vi "4.4.vi"() -> ()   [LabVIEW 2016]
panel:
  out "数组":i32[][](array[numeric])
  out "强度图":i32[][](graph)
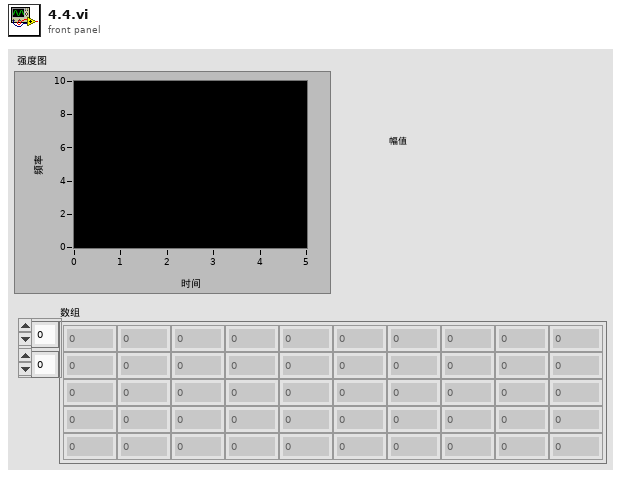
[diagram p1: front panel]
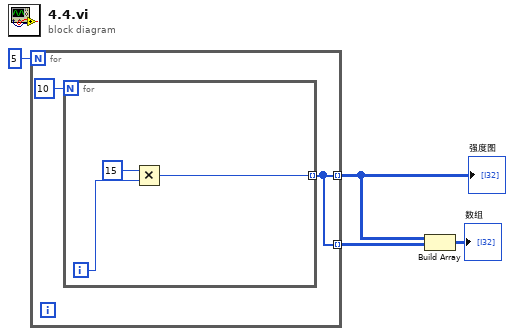
[diagram p0: block diagram]
diagram:
  n1 = for {
    N: 5 -> [_]
    tunnel: [w5] -> w2 mode=indexing
    tunnel: [w5] -> w3 mode=indexing
    n2 = for {
      N: 10 -> [_]
      tunnel: [w7] -> w5 mode=indexing
      i -> [w9]
      n3 = Multiply(x=15, y=w9) -> (x*y=w7:i32)
    }
  }
  "强度图" <- w2
  n4 = Build Array(w2, w3) -> (→"数组":i32[][][])
